vi "Periodic Tasks.vi"(8 "error in":errorcluster) -> ()   [LabVIEW 2017]
doc: "This VI runs in parallel to other tasks. It can contain as many user-defined periodic loops as you need. These can carry out PID or other sorts of timed response."
uses:
  <vilib>/Rock Robotics/WPI/Utilities/WPI_GetSetVariantRefNum.vi
  <vilib>/Rock Robotics/WPI/Ultrasonic/WPI_SonarMB1010AnalogRefNum Registry Get.vi
  <vilib>/Rock Robotics/Network Tables/NT Write Numeric Array.vi
  <vilib>/Rock Robotics/Network Tables/NT Write String Array.vi
  Robot Global Data.vi
  <vilib>/Rock Robotics/WPI/ThirdParty/Phoenix-LabVIEW/Motor Controller/Get/CTRE_Phoenix_MotorController_GetSelectedSensorData.vi
  <vilib>/Rock Robotics/Network Tables/NT Write Number.vi
  <vilib>/Rock Robotics/WPI/Ultrasonic/WPI_SonarMB1010AnalogGetRange.vi
panel:
  out "Distance":dbl
  out "Switch Pressed":bool
  out "Position (Raw Sensor Units)":i32
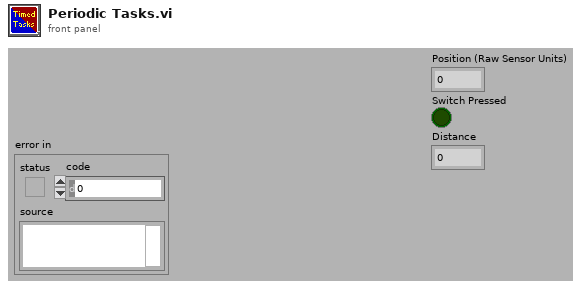
[diagram p1: front panel]
types:
  T1 = typedef "WPI_SonarMB1010AnalogDeviceRef.ctl" = cluster{"AIDeviceRef":T2, "Scaling factor (V/in)":dbl, "Average Bits":u8}
  T2 = typedef "WPI_AnalogChannelDevRef.ctl" = cluster{"DevStatus":errorcluster, "Analog Channel":T3}
  T3 = typedef "FPGA_AIChannel.ctl" = enum8{"AI 0", "AI 1", "AI 2", "AI 3", "AI MXP 0", "AI MXP 1", "AI MXP 2", "AI MXP 3", "Invalid"}
  T4 = typedef "WPI_JoystickDevRef.ctl" = cluster{"Device":T5}
  T5 = typedef "WPI_JoystickDeviceEnum.ctl" = enum16{"USB 0", "USB 1", "USB 2", "USB 3", "USB 4", "USB 5"}
  T6 = typedef "WPI_GyroDevRef.ctl" = cluster{"DevStatus":errorcluster, "Analog Channel":T3, "Gain (VoltsPerDegree/Second)":dbl, "Gyro Type":enum16{"Analog", "XRS450"}, "Handle":i32, "SPI Bus":T7, "Device Found":bool, "Sample Rate":dbl, "Calibrate On Open":bool, "Offset":dbl}
  T7 = typedef "spi_bus.ctl" = enum16{"SPI On-Board, CS0", "SPI On-Board, CS1", "SPI On-Board, CS2", "SPI On-Board, CS3", "SPI MXP", "Invalid"}
  T8 = typedef "WPI_DigitalInputDevRef.ctl" = cluster{"DevStatus":errorcluster, "DIO Channel":T9}
  T9 = typedef "FPGA_DIOChannel.ctl" = enum8{"DIO 0", "DIO 1", "DIO 2", "DIO 3", "DIO 4", "DIO 5", "DIO 6", "DIO 7", "DIO 8", "DIO 9", "DIO MXP 0", "DIO MXP 1", "DIO MXP 2", "DIO MXP 3", "DIO MXP 4", "DIO MXP 5", "DIO MXP 6", "DIO MXP 7", "DIO MXP 8", "DIO MXP 9", "DIO MXP 10", "DIO MXP 11", "DIO MXP 12", "DIO MXP 13", "DIO MXP 14", "DIO MXP 15", "SPI Port CS1", "SPI Port CS2", "SPI Port CS3", "SPI Port MISO", "SPI Port MOSI", "Invalid"}
  T10 = typedef "WPI_MotorControlDeviceRef.ctl" = cluster{"DeviceStatus":errorcluster, "Type":T11, "PWM":cluster{"PWM Channel":T12, "DeadBand":T13}, "CAN":cluster{"Device Number":u8, "SetOutput VI Ref":variant, "GetOutput VI Ref":variant, "Enable VI Ref":variant, "Disable VI Ref":variant, "Data":variant}, "Invert":bool, "DIO PWM":cluster{"PWM \"Enable\" Channel":T12, "DIOChannel":T9, "PWM Rate":dbl}}
  T11 = typedef "WPI_MotorControlType.ctl" = enum16{"PWM", "CAN", "DIO PWM"}
  T12 = typedef "FPGA_DIOPWMChannel.ctl" = enum8{"PWM 0", "PWM 1", "PWM 2", "PWM 3", "PWM 4", "PWM 5", "PWM 6", "PWM 7", "PWM 8", "PWM 9", "PWM MXP 0", "PWM MXP 1", "PWM MXP 2", "PWM MXP 3", "PWM MXP 4", "PWM MXP 5", "PWM MXP 6", "PWM MXP 7", "PWM MXP 8", "PWM MXP 9", "Invalid"}
  T13 = typedef "WPI_PWMDeadband.ctl" = cluster{"Name":string, "maxPositivePwm":i32, "minPositivePwm":i32, "centerPwm":i32, "maxNegativePwm":i32, "minNegativePwm":i32, "angularRange":u16}
  T14 = typedef "WPI_SwitchDevRef.ctl" = cluster{"DevStatus":errorcluster, "DIO Channel":T9, "CntIndex":T15, "Normally Closed":bool}
  T15 = typedef "FPGA_CounterCtrSystemIndex.ctl" = enum8{"Ctr 0", "Ctr 1", "Ctr 2", "Ctr 3", "Ctr 4", "Ctr 5", "Ctr 6", "Ctr 7", "Invalid"}
  T16 = typedef "WPI_EncoderDevRef.ctl" = cluster{"DevStatus":errorcluster, "EncoderIndex":T17, "CounterIndex":T15, "DistancePerCount":dbl, "Decoding Type":T18}
  T17 = typedef "FPGA_EncoderIdx.ctl" = enum8{"Enc 0", "Enc 1", "Enc 2", "Enc 3", "Enc 4", "Enc 5", "Enc 6", "Enc 7", "Invalid"}
  T18 = typedef "WPI_EncoderType.ctl" = enum16{"1x", "2x", "4x"}
  T19 = cluster{"JoystickDevRef":T4, "GyroDevRef":T6, "DigitalInputDevRef":T8, "SonarMB1010AnalogDevRef":T1, "PhoenixMotorControlDevRef":T10, "SwitchDevRef":T14, "EncoderDevRef":T16}
  T20 = cluster{"Yaw":dbl, "Roll":dbl, "Pitch":dbl, "Heading":dbl, "Fused Heading":dbl}
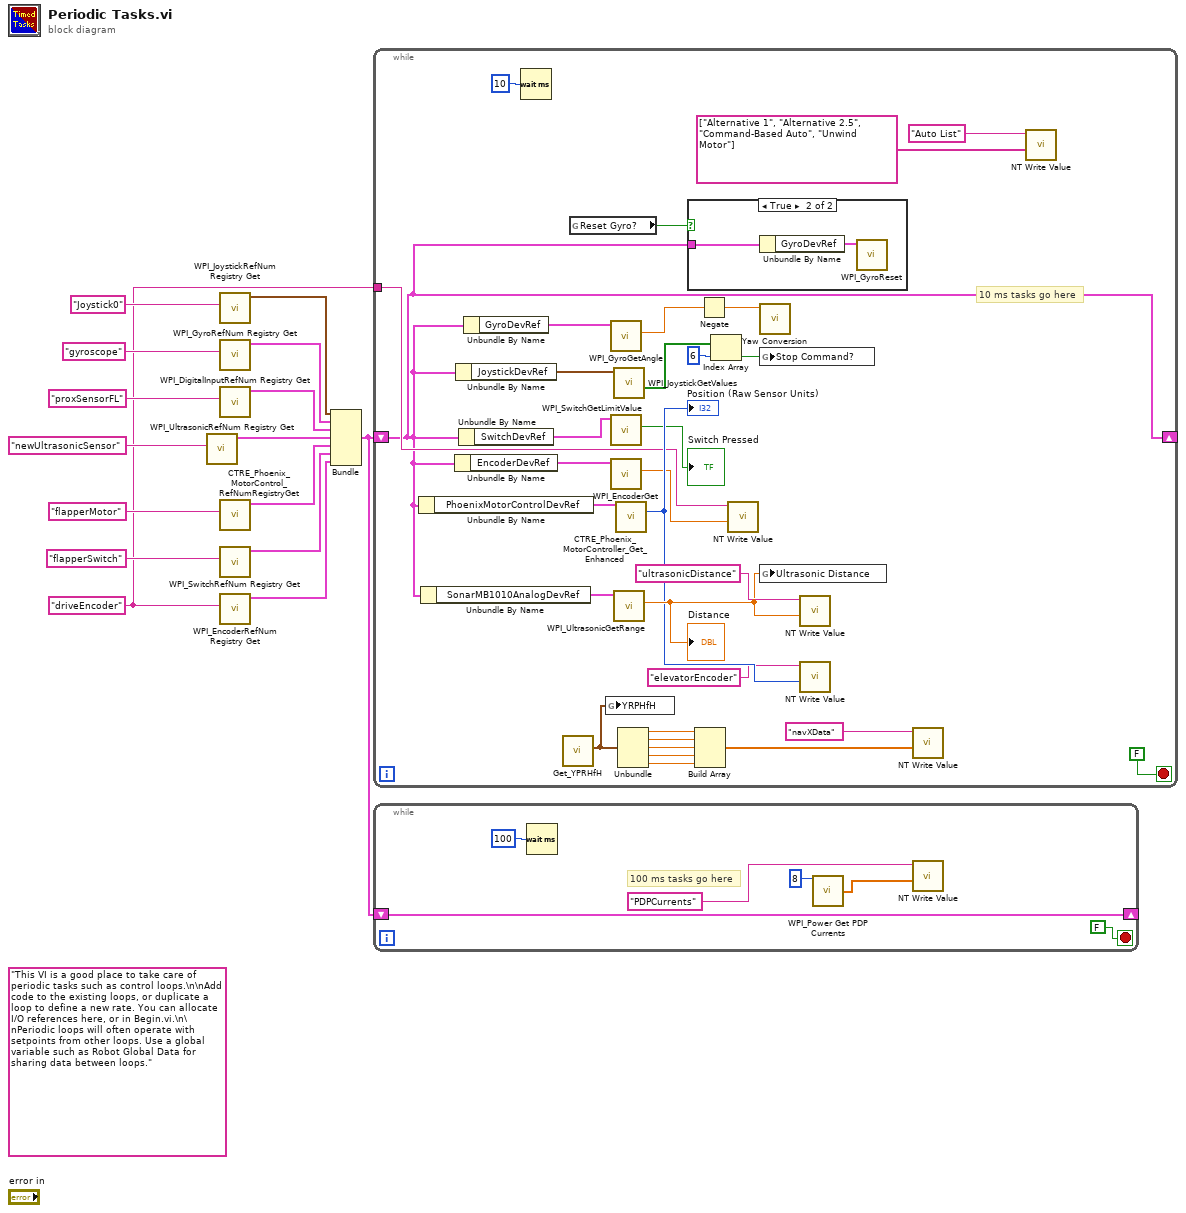
[diagram p0: block diagram]
diagram:
  w1 = "driveEncoder" ("refnum name")
  (unwired) "This VI is a good place to take care of periodic tasks such as control loops.\n\nAdd code to the existing loops, or duplicate a loop to define a new rate. You can allocate I/O references here, or in Begin.vi.\n\nPeriodic loops will often operate with setpoints from other loops. Use a global variable such as Robot Global Data for sharing data between loops."
  n1 = call-poly <vilib>:"WPI_UltrasonicRefNum Registry Get.vi"("refnum name"="newUltrasonicSensor") -> ("SonarMB1010AnalogDevRef"=w8:T1)  [unwired: 9 in, 1 out]
  n2 = call <vilib>:"WPI_JoystickRefNum Registry Get.vi"("refnum name"="Joystick0") -> ("JoystickDevRef"=w14:T4)  [unwired: 1 in, 9 out]
  n3 = call <vilib>:"WPI_GyroRefNum Registry Get.vi"("refnum name"="gyroscope") -> ("GyroDevRef"=w12:T6)  [unwired: 9 in, 1 out]
  n4 = call <vilib>:"WPI_DigitalInputRefNum Registry Get.vi"("refnum name"="proxSensorFL") -> ("DigitalInputDevRef"=w10:T8)  [unwired: 9 in, 1 out]
  n5 = call <vilib>:"CTRE_Phoenix_MotorControl_RefNumRegistryGet.vi"("refnum name"="flapperMotor") -> ("PhoenixMotorControlDevRef"=w6:T10)  [unwired: 9 in, 1 out]
  n6 = call <vilib>:"WPI_SwitchRefNum Registry Get.vi"("refnum name"="flapperSwitch") -> ("SwitchDevRef"=w3:T14)  [unwired: 9 in, 1 out]
  n7 = call <vilib>:"WPI_EncoderRefNum Registry Get.vi"("refnum name"=w1) -> ("EncoderDevRef"=w2:T16)  [unwired: 9 in, 1 out]
  n8 = Bundle("JoystickDevRef"=w14, "GyroDevRef"=w12, "DigitalInputDevRef"=w10, "SonarMB1010AnalogDevRef"=w8, "PhoenixMotorControlDevRef"=w6, "SwitchDevRef"=w3, "EncoderDevRef"=w2) -> (w13:T19)  [unwired: 1 out]
  n9 = while {
    shift-right: [w17] -> _
    shift-left: w13 -> [w17]
    tunnel: w1 -> [w19]
    stop <- FALSE stop-if-true
    # "10 ms tasks go here"
    n10 = Unbundle By Name(w17) -> ("PhoenixMotorControlDevRef"=w26:T10)
    n11 = Unbundle By Name(w17) -> ("SonarMB1010AnalogDevRef"=w38:T1)
    n12 = Unbundle By Name(w17) -> ("EncoderDevRef"=w16:T16)
    n13 = Unbundle By Name(w17) -> ("JoystickDevRef"=w45:T4)
    n14 = Unbundle By Name(w17) -> ("SwitchDevRef"=w23:T14)
    n15 = Unbundle By Name(w17) -> ("GyroDevRef"=w40:T6)
    n16 = Wait (ms)(milliseconds to wait=u32 10) -> ()  [unwired: 1 out]
    n17 = call <vilib>:"Get_YPRHfH.vi"() -> ("YRPHfH"=w33:T20)  [unwired: 11 in]
    n18 = global read "Robot Global Data.vi" "Reset Gyro?"() -> (w35:bool)
    n19 = global write "Robot Global Data.vi" "YRPHfH"(w33) -> ()
    n20 = call <vilib>:"WPI_GyroGetAngle.vi"("GyroDevRef"=w40) -> ("Angle"=w41:dbl)  [unwired: 6 in, 4 out]
    n21 = call <vilib>:"WPI_SwitchGetLimitValue.vi"("SwitchDevRef"=w23) -> ("Switch Pressed"=→"Switch Pressed":bool)  [unwired: 8 in, 2 out]
    n22 = call <vilib>:"WPI_EncoderGet.vi"("EncoderDevRef"=w16) -> ("Distance"=w18:dbl)  [unwired: 5 in, 5 out]
    n23 = call <vilib>:"WPI_JoystickGetValues.vi"("JoystickDevRef"=w45) -> ("Buttons"=w44:bool[])  [unwired: 6 in, 4 out]
    n24 = call-poly <vilib>:"WPI_UltrasonicGetRange.vi"("SonarMB1010AnalogDevRef"=w38) -> ("Distance"=w36:dbl)  [unwired: 8 in, 2 out]
    "Distance" <- w36
    n25 = call-poly <vilib>:"CTRE_Phoenix_MotorController_Get_Enhanced.vi"("PhoenixMotorControlDevRef"=w26) -> ("Position (Raw Sensor Units)"=w25:i32)  [unwired: 11 in, 3 out]
    "Position (Raw Sensor Units)" <- w25
    n26 = Unbundle(w33) -> ("Yaw"=w32:dbl, "Roll"=w31:dbl, "Pitch"=w30:dbl, "Heading"=w29:dbl, "Fused Heading"=w28:dbl)
    n27 = case shown="True" w35 {
      tunnel: w17 -> [_ w48]
      frame False {
      }
      frame True {
        n28 = Unbundle By Name(w48) -> ("GyroDevRef"=w49:T6)
        n29 = call <vilib>:"WPI_GyroReset.vi"("GyroDevRef"=w49) -> ()  [unwired: 9 in, 2 out]
      }
    }
    n30 = Build Array(w32, w31, w30, w29, w28) -> (w27:dbl[])
    n31 = Negate(x=w41) -> (-x=w42:dbl)
    n32 = Index Array(array=w44, index=6) -> (element=w34:bool)
    n33 = call-poly <vilib>:"NT Write Value.vi"("Numeric"=w18, "Name"=w19) -> ()  [unwired: 9 in, 1 out]
    n34 = call "Yaw Conversion.vi"("Input"=w42) -> ()  [unwired: 10 in, 1 out]
    n35 = global write "Robot Global Data.vi" "Stop Command?"(w34) -> ()
    n36 = global write "Robot Global Data.vi" "Ultrasonic Distance"(w36) -> ()
    n37 = call-poly <vilib>:"NT Write Value.vi"("Numeric"=w36, "Name"="ultrasonicDistance") -> ()  [unwired: 9 in, 1 out]
    n38 = call-poly <vilib>:"NT Write Value.vi"("Numeric"=w25, "Name"="elevatorEncoder") -> ()  [unwired: 9 in, 1 out]
    n39 = call-poly <vilib>:"NT Write Value.vi"("Numeric Array"=w27, "Name"="navXData") -> ()  [unwired: 9 in, 1 out]
    n40 = call-poly <vilib>:"NT Write Value.vi"("String Array"=string[] ["Alternative 1", "Alternative 2.5", "Command-Based Auto", "Unwind Motor"], "Name"="Auto List") -> ()  [unwired: 9 in, 1 out]
  }
  n41 = while {
    shift-right: [w50] -> _
    shift-left: w13 -> [w50]
    stop <- FALSE stop-if-true
    # "100 ms tasks go here"
    n42 = Wait (ms)(milliseconds to wait=u32 100) -> ()  [unwired: 1 out]
    n43 = call <vilib>:"WPI_Power Get PDP Currents.vi"("Power Distribution Panel (0)"=u8 8) -> ("all currents (A)"=w52:dbl[])  [unwired: 12 in, 2 out]
    n44 = call-poly <vilib>:"NT Write Value.vi"("Numeric Array"=w52, "Name"="PDPCurrents") -> ()  [unwired: 9 in, 1 out]
  }
